vi "Actor Core.vi"(8 "error in":errorcluster, 11 "Actor_Controller_Template in":refnum<class "Actor_Controller_Template.lvclass">) -> (0 "error out":errorcluster, 3 "Actor out":refnum<class "Actor.lvclass">)   [LabVIEW 2020, in "Actor_Controller_Template.lvlib" / "Actor_Controller_Template.lvclass"]
doc: "(<B>Filename</B>: Actor Framework.lvlib:Actor.lvclass:Actor Core.vi)\n\nReceives messages to the actor, reacts to them, and initiates any error handling that may shut the actor down.\n\nDescendant classes may override this VI to append parallel tasks for the actor to complete while it handles messages. Overrides use the Call Parent Class Method node."
uses:
  Actor_Controller_Template.lvclass
  C:/Program Files/National Instruments/LabVIEW 2020/vi.lib/ActorFramework/Actor/Actor.lvclass
  <vilib>/ActorFramework/Actor/Actor.lvclass
  Actor_UI_Template/Actor_UI_Template/Actor_UI_Template.lvclass
  Actor_Controller_Template.lvclass/Actor_Controller_Template.ctl
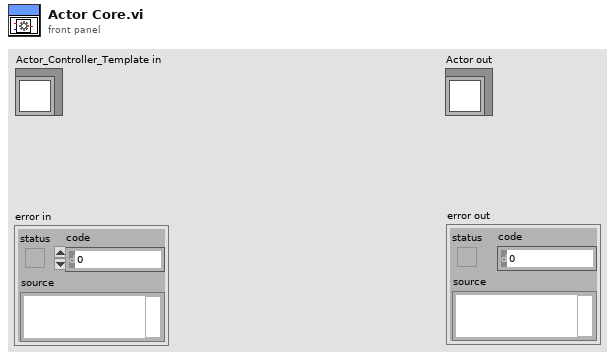
[diagram p1: front panel]
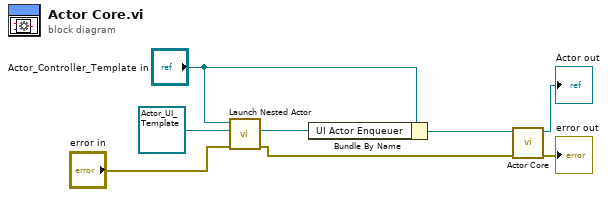
[diagram p0: block diagram]
diagram:
  n1 = call <vilib>:"Launch Nested Actor.vi"("error in (no error)"="error in", "Nested Actor"=refnum<class "Actor_UI_Template.lvclass"> refnum ("Actor_UI_Template.lvlib:Actor_UI_Template.lvclass"), "Caller Actor in"="Actor_Controller_Template in") -> ("error out"=w2:errorcluster, "Nested Actor's Enqueuer"=w1:refnum<class "Message Enqueuer.lvclass">)  [unwired: 6 in, 1 out]
  n2 = Bundle By Name(cluster="Actor_Controller_Template in", "UI Actor Enqueuer"=w1) -> (w4:refnum<class "Actor_Controller_Template.lvclass">)
  n3 = call-parent "Actor Core.vi"("error in"=w2, "Actor in"=w4) -> ("error out"=→"error out":errorcluster, "Actor out"=→"Actor out":refnum<class "Actor.lvclass">)  [unwired: 8 in]
